vi "Encapsulate TCP Payload.vi"(5 "task_id":string, 6 "source_id":u32, 7 "target_node":u32, 8 "error in (no error)":errorcluster, 9 "type":string, 10 "Encapsulated Payload":u8[](array[numeric])) -> (0 "error out":errorcluster, 2 "TCP Payload":string)   [LabVIEW 2020, in "Vecto.lvlib"]
uses:
  Vecto.lvlib
  SequenceCountService/SequenceCountService.lvclass
  proto/TcpPayload/Data.ctl
  proto/TcpPayload/TcpPayload.lvlib
panel:
  in  "SequenceCountService":refnum<class "SequenceCountService.lvclass">
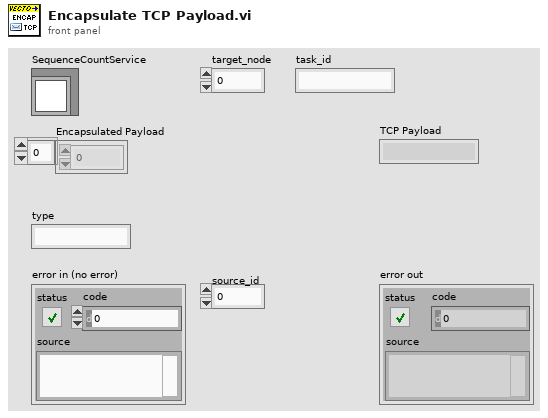
[diagram p1: front panel]
types:
  T1 = typedef "TcpPayload.lvlib/Data.ctl" = cluster{"target_node":u32, "source_id":u32, "sequence":u32, "timestamp":u64, "type":string, "task_id":string, "payload":u8[]}
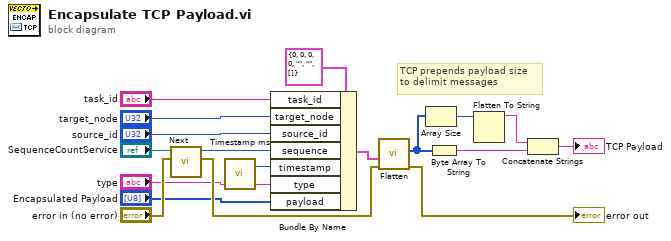
[diagram p0: block diagram]
diagram:
  # "TCP prepends payload size to delimit messages"
  n1 = call "Next.vi"("error in (no error)"="error in (no error)", "SequenceCountService in"="SequenceCountService") -> ("error out"=w18:errorcluster, "Sequence"=w10:u32)  [unwired: 8 in]
  n2 = call "Timestamp ms.vi"() -> ("Timestamp ms"=w12:u64)  [unwired: 7 in]
  n3 = Bundle By Name(cluster=T1 {"target_node"=0, "source_id"=0, "sequence"=0, "timestamp"=0, "type"="", "task_id"="", "payload"=[]} ("TcpPayload"), "task_id"="task_id", "target_node"="target_node", "source_id"="source_id", "sequence"=w10, "timestamp"=w12, "type"="type", "payload"="Encapsulated Payload") -> (w9:T1)
  n4 = call "Flatten.vi"("error in"=w18, "Data"=w9) -> ("error out"=→"error out":errorcluster, "Buffer"=w6:u8[])  [unwired: 8 in]
  n5 = Array Size(array=w6) -> (size(s)=w5:i32)
  n6 = Byte Array To String(unsigned byte array=w6) -> (string=w7:string)
  n7 = Flatten To String(anything=w5) -> (data string=w3:string)  [unwired: 3 in, 2 out]
  n8 = Concatenate Strings(w3, w7) -> (→"TCP Payload":string)
